vi "Set FPGA target.vi"(8 "error in (no error)":errorcluster, 10 "Number of bits":i32, 11 "Boolean array":bool[](array[boolean])) -> (0 "error out":errorcluster)   [LabVIEW 2013]
uses:
  <vilib>/DAQmx/write.llb/DAQmx Write (Digital Bool 1Line 1Point).vi
  <vilib>/DAQmx/miscellaneous.llb/DAQmx Fill In Error Info.vi
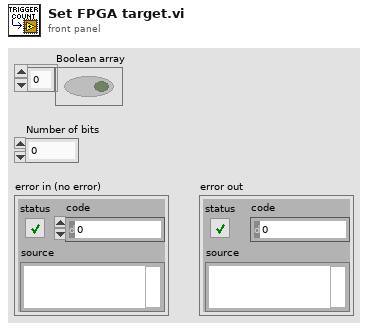
[diagram p1: front panel]
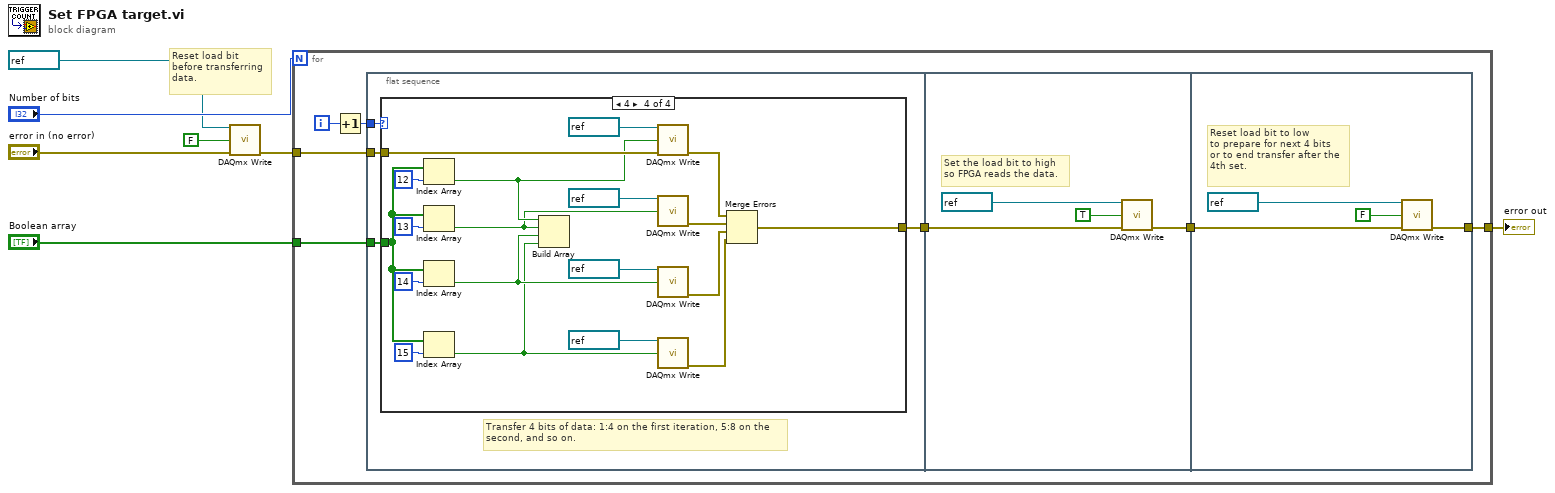
[diagram p0: block diagram]
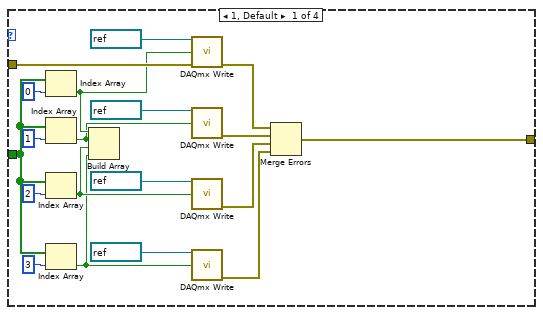
[diagram p2: hidden frame]
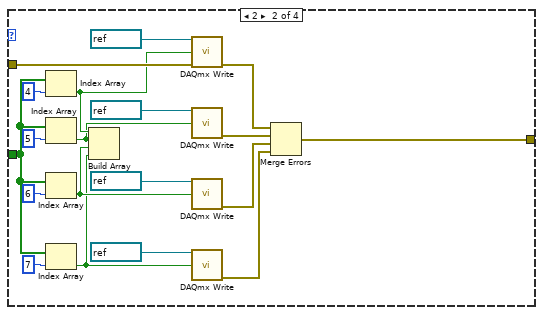
[diagram p3: hidden frame]
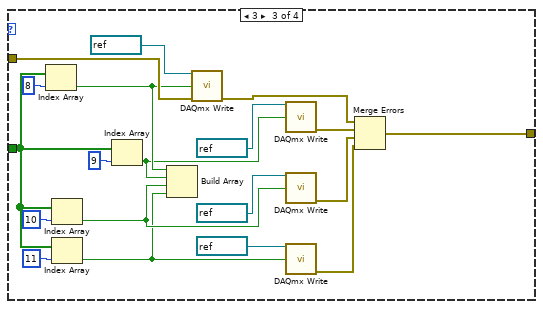
[diagram p4: hidden frame]
diagram:
  # "Reset load bit\nbefore transferring\ndata."
  n1 = call-poly <vilib>:"DAQmx Write.vi"("task/channels in"=refnum<k21> "BIT5", "data"=FALSE, "error in"="error in (no error)") -> ("error out"=w1:errorcluster)  [unwired: 10 in, 2 out]
  n2 = for {
    N: "Number of bits" -> [_]
    tunnel: "Boolean array" -> [w11]
    tunnel: w1 -> [w13]
    tunnel: [w8] -> w7
    i -> [w14]
    n3 = Increment(x=w14) -> (x+1=w12:i32)
    n4 = flat-sequence {
      tunnel: w13 -> [w18]
      tunnel: w12 -> [w17]
      tunnel: w11 -> [w16]
      tunnel: [w15] -> w10
      tunnel: w10 -> [w96]
      tunnel: [w95] -> w9
      tunnel: w9 -> [w100]
      tunnel: [w99] -> w8
      frame #0 {
        # "Transfer 4 bits of data: 1:4 on the first iteration, 5:8 on the\nsecond, and so on."
        n5 = case shown="4" w17 {
          tunnel: w16 -> [w25 w44 w63 w82]
          tunnel: w18 -> [w24 w43 w62 w81]
          tunnel: [w23 w42 w61 w80] -> w15
          frame 1, Default {
            n6 = Index Array(array=w25, index=0) -> (element=w22:bool)
            n7 = Index Array(array=w25, index=1) -> (element=w21:bool)
            n8 = Index Array(array=w25, index=2) -> (element=w20:bool)
            n9 = Index Array(array=w25, index=3) -> (element=w19:bool)
            n10 = Build Array(w22, w21, w20, w19) -> ()  [unwired: 1 out]
            n11 = call-poly <vilib>:"DAQmx Write.vi"("task/channels in"=refnum<k21> "BIT1", "data"=w22, "error in"=w24) -> ("error out"=w33:errorcluster)  [unwired: 10 in, 2 out]
            n12 = call-poly <vilib>:"DAQmx Write.vi"("task/channels in"=refnum<k21> "BIT2", "data"=w21) -> ("error out"=w32:errorcluster)  [unwired: 11 in, 2 out]
            n13 = call-poly <vilib>:"DAQmx Write.vi"("task/channels in"=refnum<k21> "BIT3", "data"=w20) -> ("error out"=w31:errorcluster)  [unwired: 11 in, 2 out]
            n14 = call-poly <vilib>:"DAQmx Write.vi"("task/channels in"=refnum<k21> "BIT4", "data"=w19) -> ("error out"=w30:errorcluster)  [unwired: 11 in, 2 out]
            n15 = Merge Errors(w33, w32, w31, w30) -> (w23:errorcluster)
          }
          frame 2 {
            n16 = Index Array(array=w44, index=4) -> (element=w41:bool)
            n17 = Index Array(array=w44, index=5) -> (element=w40:bool)
            n18 = Index Array(array=w44, index=6) -> (element=w39:bool)
            n19 = Index Array(array=w44, index=7) -> (element=w38:bool)
            n20 = Build Array(w41, w40, w39, w38) -> ()  [unwired: 1 out]
            n21 = call-poly <vilib>:"DAQmx Write.vi"("task/channels in"=refnum<k21> "BIT1", "data"=w41, "error in"=w43) -> ("error out"=w52:errorcluster)  [unwired: 10 in, 2 out]
            n22 = call-poly <vilib>:"DAQmx Write.vi"("task/channels in"=refnum<k21> "BIT2", "data"=w40) -> ("error out"=w51:errorcluster)  [unwired: 11 in, 2 out]
            n23 = call-poly <vilib>:"DAQmx Write.vi"("task/channels in"=refnum<k21> "BIT3", "data"=w39) -> ("error out"=w50:errorcluster)  [unwired: 11 in, 2 out]
            n24 = call-poly <vilib>:"DAQmx Write.vi"("task/channels in"=refnum<k21> "BIT4", "data"=w38) -> ("error out"=w49:errorcluster)  [unwired: 11 in, 2 out]
            n25 = Merge Errors(w52, w51, w50, w49) -> (w42:errorcluster)
          }
          frame 3 {
            n26 = Index Array(array=w63, index=8) -> (element=w60:bool)
            n27 = Index Array(array=w63, index=10) -> (element=w58:bool)
            n28 = Index Array(array=w63, index=11) -> (element=w57:bool)
            n29 = Index Array(array=w63, index=9) -> (element=w59:bool)
            n30 = Build Array(w60, w59, w58, w57) -> ()  [unwired: 1 out]
            n31 = call-poly <vilib>:"DAQmx Write.vi"("task/channels in"=refnum<k21> "BIT1", "data"=w60, "error in"=w62) -> ("error out"=w71:errorcluster)  [unwired: 10 in, 2 out]
            n32 = call-poly <vilib>:"DAQmx Write.vi"("task/channels in"=refnum<k21> "BIT2", "data"=w59) -> ("error out"=w70:errorcluster)  [unwired: 11 in, 2 out]
            n33 = call-poly <vilib>:"DAQmx Write.vi"("task/channels in"=refnum<k21> "BIT3", "data"=w58) -> ("error out"=w69:errorcluster)  [unwired: 11 in, 2 out]
            n34 = call-poly <vilib>:"DAQmx Write.vi"("task/channels in"=refnum<k21> "BIT4", "data"=w57) -> ("error out"=w68:errorcluster)  [unwired: 11 in, 2 out]
            n35 = Merge Errors(w71, w70, w69, w68) -> (w61:errorcluster)
          }
          frame 4 {
            n36 = Index Array(array=w82, index=12) -> (element=w79:bool)
            n37 = Index Array(array=w82, index=13) -> (element=w78:bool)
            n38 = Index Array(array=w82, index=14) -> (element=w77:bool)
            n39 = Index Array(array=w82, index=15) -> (element=w76:bool)
            n40 = Build Array(w79, w78, w77, w76) -> ()  [unwired: 1 out]
            n41 = call-poly <vilib>:"DAQmx Write.vi"("task/channels in"=refnum<k21> "BIT1", "data"=w79, "error in"=w81) -> ("error out"=w90:errorcluster)  [unwired: 10 in, 2 out]
            n42 = call-poly <vilib>:"DAQmx Write.vi"("task/channels in"=refnum<k21> "BIT2", "data"=w78) -> ("error out"=w89:errorcluster)  [unwired: 11 in, 2 out]
            n43 = call-poly <vilib>:"DAQmx Write.vi"("task/channels in"=refnum<k21> "BIT3", "data"=w77) -> ("error out"=w88:errorcluster)  [unwired: 11 in, 2 out]
            n44 = call-poly <vilib>:"DAQmx Write.vi"("task/channels in"=refnum<k21> "BIT4", "data"=w76) -> ("error out"=w87:errorcluster)  [unwired: 11 in, 2 out]
            n45 = Merge Errors(w90, w89, w88, w87) -> (w80:errorcluster)
          }
        }
      }
      frame #1 {
        # "Set the load bit to high\nso FPGA reads the data."
        n46 = call-poly <vilib>:"DAQmx Write.vi"("task/channels in"=refnum<k21> "BIT5", "data"=TRUE, "error in"=w96) -> ("error out"=w95:errorcluster)  [unwired: 10 in, 2 out]
      }
      frame #2 {
        # "Reset load bit to low\nto prepare for next 4 bits\nor to end transfer after the\n4th set."
        n47 = call-poly <vilib>:"DAQmx Write.vi"("task/channels in"=refnum<k21> "BIT5", "data"=FALSE, "error in"=w100) -> ("error out"=w99:errorcluster)  [unwired: 10 in, 2 out]
      }
    }
  }
  "error out" <- w7
